vi "ATF Pump-Device List.vi"(9 "output cluster":T1, 10 "DL":string, 11 "Enum":enum16{"Write", "Read"}(ring)) -> (1 "output cluster 2":T1, 2 "DL 2":string)   [LabVIEW 2022 SP3]
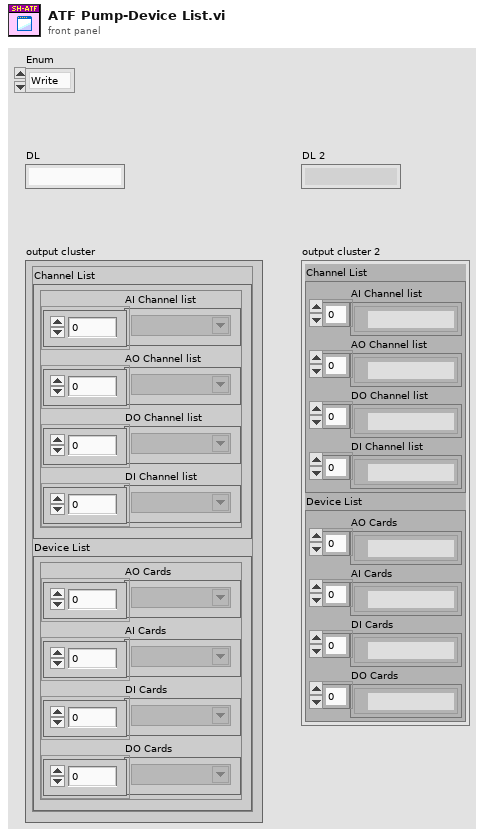
[diagram p1: front panel]
types:
  T1 = cluster{"Channel List":cluster{"AI Channel list":tag[], "AO Channel list":tag[], "DO Channel list ":tag[], "DI Channel list":tag[]}, "Device List":cluster{"AO Cards":tag[], "AI Cards":tag[], "DI Cards":tag[], "DO Cards":tag[]}}
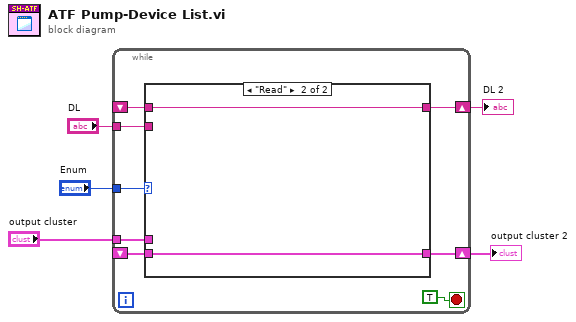
[diagram p0: block diagram]
diagram:
  n1 = while {
    tunnel: "Enum" -> [w12]
    tunnel: "output cluster" -> [w11]
    shift-right: [w10] -> w3
    shift-left: _ -> [w9]
    tunnel: "DL" -> [w8]
    shift-right: [w7] -> w1
    shift-left: _ -> [w6]
    stop <- TRUE stop-if-true
    n2 = case shown="\"Read\"" w12 {
      tunnel: [w15 w17] -> w10
      tunnel: w11 -> [w15 _]
      tunnel: w9 -> [_ w17]
      tunnel: w8 -> [w14 _]
      tunnel: [w14 w16] -> w7
      tunnel: w6 -> [_ w16]
      frame "Write", Default {
      }
      frame "Read" {
      }
    }
  }
  "output cluster 2" <- w3
  "DL 2" <- w1
